vi "DP41 Raw Serial Read Write.vi"(7 "Read Only?":bool, 8 "error in (no error)":errorcluster, 10 "Command Write":string, 11 "VISA Refnum in":refnum<visa-resource-name>) -> (0 "error out":errorcluster, 2 "Data Stream":string, 3 "VISA Refnum out":refnum<visa-resource-name>)   [LabVIEW 2016]
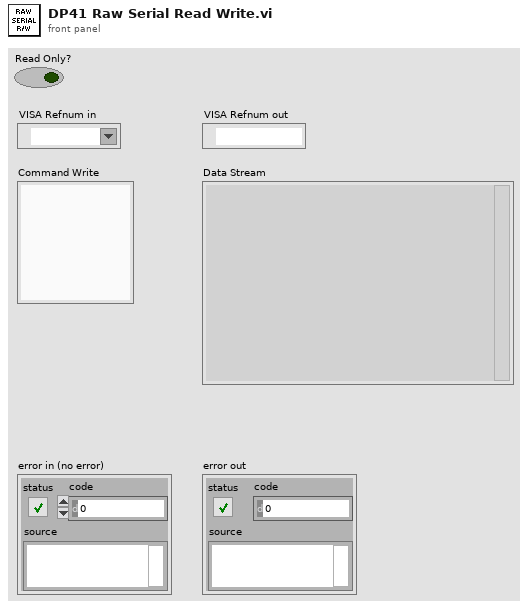
[diagram p1: front panel]
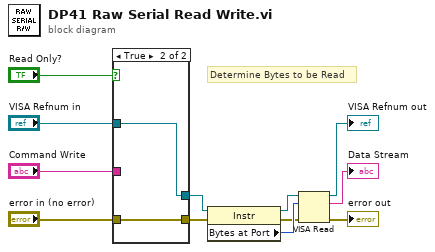
[diagram p0: block diagram]
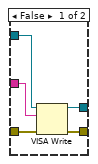
[diagram p2: hidden frame]
diagram:
  # "Determine Bytes to be Read"
  n1 = case shown="True" "Read Only?" {
    tunnel: [w17 w19] -> w10
    tunnel: [w16 w18] -> w8
    tunnel: "Command Write" -> [w15 _]
    tunnel: "VISA Refnum in" -> [w14 w18]
    tunnel: "error in (no error)" -> [w13 w19]
    frame False {
      n2 = VISA Write(VISA resource name=w14, write buffer=w15, error in (no error)=w13) -> (VISA resource name out=w16:refnum<visa-resource-name>, error out=w17:errorcluster)  [unwired: 1 out]
    }
    frame True {
    }
  }
  n3 = property class="Instr"(reference=w8, error in=w10) -> (reference out=w9:refnum<visa-resource-name>, error out=w11:errorcluster, "Bytes at Port"=w12:u32)
  n4 = VISA Read(VISA resource name=w9, byte count=w12, error in (no error)=w11) -> (VISA resource name out=→"VISA Refnum out":refnum<visa-resource-name>, read buffer=→"Data Stream":string, error out=→"error out":errorcluster)  [unwired: 1 out]
